vi "SetBoolValue.vi"(3 "error in (no error)":errorcluster, 4 "bValue":bool, 5 "strName":string, 6 "nInputHandle":u64) -> (0 "error out":errorcluster, 1 "GX_STATUS":i32, 2 "nOutputHandle":u64)   [LabVIEW 2016, in "GxLVLib.lvlib"]
uses:
  GxLVLib.lvlib
  GxIAPI.dll
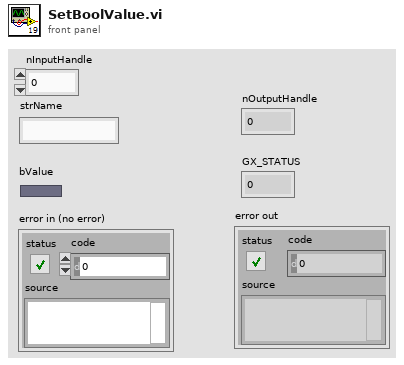
[diagram p1: front panel]
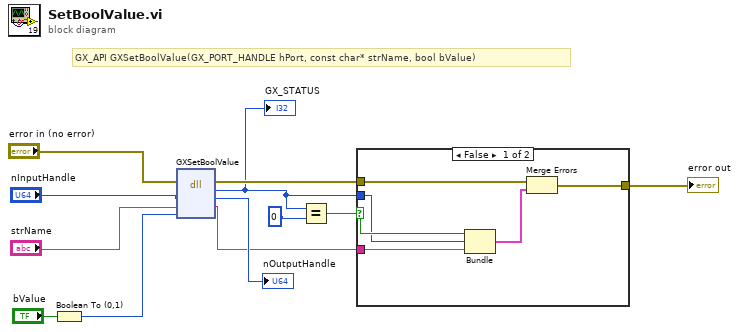
[diagram p0: block diagram]
diagram:
  # "GX_API GXSetBoolValue(GX_PORT_HANDLE hPort, const char* strName, bool bValue)"
  n1 = Boolean To (0,1)(Boolean="bValue") -> (0, 1=w11:i16)
  n2 = dll-call lib="GxIAPI.dll" fn="GXSetBoolValue"(error in="error in (no error)", "phDevice"="nInputHandle", "strName"="strName", "bValue"=w11) -> (error out=w9:errorcluster, "GX_STATUS"=w5:i64, "phDevice"=→"nOutputHandle":i32, "strName"=w6:string)  [unwired: 3 in, 1 out]
  "GX_STATUS" <- w5
  n3 = Equal?(x=w5, y=0) -> (x = y?=w8:bool)
  n4 = case shown="False" w8 {
    selector: w8 -> [w15 _]
    tunnel: w9 -> [w18 w19]
    tunnel: [w17 w19] -> w4
    tunnel: w5 -> [w14 _]
    tunnel: w6 -> [w13 _]
    frame False {
      n5 = Bundle(w15, "GX_STATUS"=w14, "strName"=w13) -> (w16:cluster{bool, "GX_STATUS":i64, "strName":string})  [unwired: 1 in]
      n6 = Merge Errors(w18, w16) -> (w17:errorcluster)
    }
    frame True {
    }
  }
  "error out" <- w4
